vi "Teleop.vi"(10 "Match Info":T1={"Autonomous Elapsed Seconds"=0.0, "TeleOp Elapsed Seconds"=0.0, "Disabled Elapsed Seconds"=0.0, "Visited Autonomous"=FALSE, "Visited TeleOp"=FALSE, "Visited Disabled"=FALSE, "Autonomous Settings"={"Autonomous Style"=enum."Independent", "VI Refnum"=refnum}}, 11 "Call Context":T2) -> ()   [LabVIEW 2019]
doc: "This VI is called for each enabled TeleOp packet received from the DS. It is typically used to read from joysticks and other inputs and update I/O or setpoints for timed control loops. It should complete and return within 20 milliseconds or risk missing DS packets."
uses:
  <vilib>/Rock Robotics/WPI/DriverStation/WPI_DriverStationDerivedRobotMode.ctl
  <vilib>/Rock Robotics/WPI/DriverStation/WPI_DriverStationMatch Info.ctl
  <vilib>/Rock Robotics/WPI/Utilities/WPI_GetSetVariantRefNum.vi
  <vilib>/Rock Robotics/Network Tables/NT Write Boolean Array.vi
  <vilib>/Rock Robotics/Network Tables/NT Write Numeric Array.vi
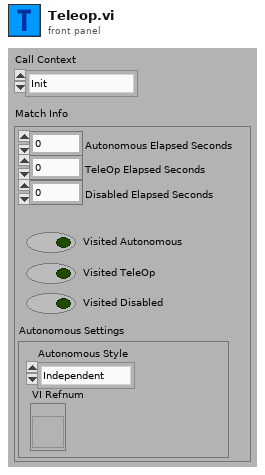
[diagram p1: front panel]
types:
  T1 = typedef "WPI_DriverStationMatch Info.ctl" = cluster{"Autonomous Elapsed Seconds":dbl, "TeleOp Elapsed Seconds":dbl, "Disabled Elapsed Seconds":dbl, "Visited Autonomous":bool, "Visited TeleOp":bool, "Visited Disabled":bool, "Autonomous Settings":cluster{"Autonomous Style":enum16{"Iterative", "Independent"}, "VI Refnum":refnum<vi>}}
  T2 = typedef "WPI_DriverStationDerivedRobotMode.ctl" = enum16{"Init", "Execute", "Stop"}
  T3 = typedef "WPI_JoystickDevRef.ctl" = cluster{"Device":T4}
  T4 = typedef "WPI_JoystickDeviceEnum.ctl" = enum16{"USB 0", "USB 1", "USB 2", "USB 3", "USB 4", "USB 5"}
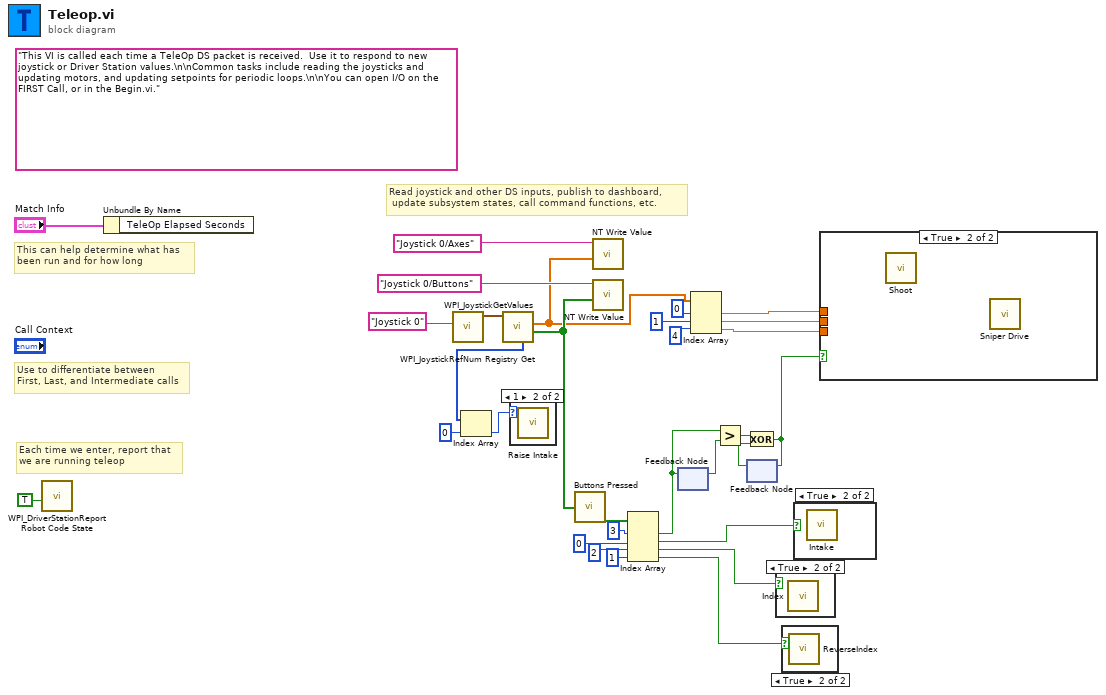
[diagram p0: block diagram]
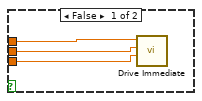
[diagram p6: hidden frame]
diagram:
  (unwired) "This VI is called each time a TeleOp DS packet is received.  Use it to respond to new joystick or Driver Station values.\n\nCommon tasks include reading the joysticks and updating motors, and updating setpoints for periodic loops.\n\nYou can open I/O on the FIRST Call, or in the Begin.vi."
  # "Read joystick and other DS inputs, publish to dashboard,\n update subsystem states, call command functions, etc."
  # "Each time we enter, report that\nwe are running teleop"
  # "Use to differentiate between\nFirst, Last, and Intermediate calls"
  # "This can help determine what has\nbeen run and for how long"
  n1 = call <vilib>:"WPI_DriverStationReport Robot Code State.vi"("TeleOp"=TRUE ("Autonomous")) -> ()  [unwired: 10 in, 1 out]
  n2 = Unbundle By Name("Match Info") -> ()  [unwired: 1 out]
  n3 = call <vilib>:"WPI_JoystickRefNum Registry Get.vi"("refnum name"="Joystick 0") -> ("JoystickDevRef"=w27:T3)  [unwired: 1 in, 9 out]
  n4 = call <vilib>:"WPI_JoystickGetValues.vi"("JoystickDevRef"=w27) -> ("Buttons"=w24:bool[], "Axes"=w19:dbl[], "POVs"=w3:i16[])  [unwired: 6 in, 2 out]
  n5 = Index Array(array=w3, index=0) -> (element=w1:i16)
  n6 = case shown="1" w1 {
    frame 0, Default {
    }
    frame 1 {
      n7 = call "Raise Intake.vi"() -> ()  [unwired: 11 in, 1 out]
    }
  }
  n8 = call "Buttons Pressed.vi"("Button Values"=w24) -> ("Button Presses"=w26:bool[])
  n9 = call-poly <vilib>:"NT Write Value.vi"("Numeric Array"=w19, "Name"="Joystick 0/Axes") -> ()  [unwired: 9 in, 1 out]
  n10 = call-poly <vilib>:"NT Write Value.vi"("Boolean Array"=w24, "Name"="Joystick 0/Buttons") -> ()  [unwired: 9 in, 1 out]
  n11 = Index Array(array=w26, index #1=3 ("index"), index #2=0 ("index"), index #3=2 ("index"), index #4=1 ("index")) -> (element #1=w10:bool, element #2=w9:bool, element #3=w7:bool, element #4=w4:bool)
  n12 = feedback #1() -> (w15:bool)  [unwired: 1 in]
  n13 = feedback-in #1(w10) -> ()
  n14 = Index Array(array=w19, index #1=0 ("index"), index #2=1 ("index"), index #3=4 ("index")) -> (element #1=w18:dbl, element #2=w17:dbl, element #3=w16:dbl)
  n15 = Greater?(x=w10, y=w15) -> (0:w14:bool)
  n16 = feedback #2() -> (w13:bool)  [unwired: 1 in]
  n17 = Exclusive Or(1:w13, 2:w14) -> (0:w12:bool)
  n18 = feedback-in #2(w12) -> ()
  n19 = case shown="True" w7 {
    frame False {
    }
    frame True {
      n20 = call "Index.vi"() -> ()  [unwired: 11 in, 1 out]
    }
  }
  n21 = case shown="True" w4 {
    frame False {
    }
    frame True {
      n22 = call "ReverseIndex.vi"() -> ()  [unwired: 11 in, 1 out]
    }
  }
  n23 = case shown="True" w9 {
    frame False {
    }
    frame True {
      n24 = call "Intake.vi"() -> ()  [unwired: 11 in, 1 out]
    }
  }
  n25 = case shown="True" w12 {
    tunnel: w18 -> [w33 _]
    tunnel: w17 -> [w32 _]
    tunnel: w16 -> [w31 _]
    frame False {
      n26 = call "Drive Immediate.vi"("Right joystick x"=w31, "Left joystick y"=w32, "Left joystick x"=w33) -> ()  [unwired: 8 in, 1 out]
    }
    frame True {
      n27 = call "Shoot.vi"() -> ()  [unwired: 11 in, 1 out]
      n28 = call "Sniper Drive.vi"() -> ()  [unwired: 11 in, 1 out]
    }
  }
